vi "SetRef.vi"(8 "error in (no error)":errorcluster, 10 "Set External":bool, 11 "NetA_RSZVL in":refnum<class "NetA_RSZVL.lvclass">) -> (0 "error out":errorcluster, 3 "NetA_RSZVL out":refnum<class "NetA_RSZVL.lvclass">)   [LabVIEW 2014, in "NetA_RSZVL.lvclass"]
uses:
  NetA_RSZVL.lvclass
  NetA_RSZVL.lvclass/NetA_RSZVL.ctl
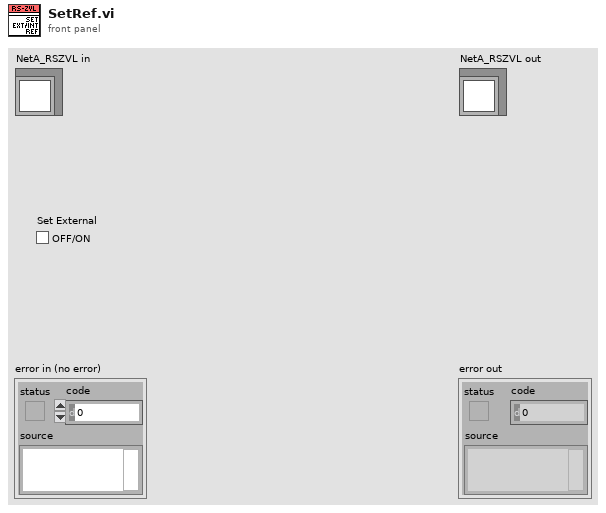
[diagram p1: front panel]
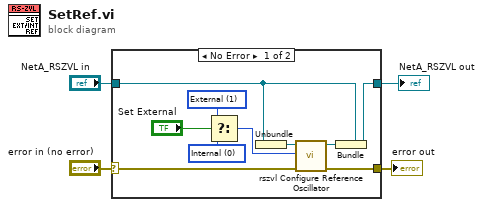
[diagram p0: block diagram]
diagram:
  n1 = case shown="No Error" "error in (no error)" {
    selector: "error in (no error)" -> [w14 w15]
    tunnel: "NetA_RSZVL in" -> [w8 w16]
    tunnel: [w6 w15] -> w2
    tunnel: [w5 w16] -> w1
    frame No Error {
      w11 = 0 items=["Internal", "External"] ("Reference (Internal)")
      w12 = 1 items=["Internal", "External"] ("Reference (Internal)")
      n2 = Select(t=w12, s="Set External", f=w11) -> (s? t:f=w10:i32)
      n3 = Unbundle(w8) -> (w9:refnum<visa-resource-name>)
      n4 = call "rszvl Configure Reference Oscillator.vi"("error in (no error)"=w14, "Reference (Internal)"=w10, "VISA resource name"=w9) -> ("error out"=w6:errorcluster, "VISA resource name out"=w7:refnum<visa-resource-name>)  [unwired: 7 in]
      n5 = Bundle(cluster=w8, w7) -> (w5:refnum<class "NetA_RSZVL.lvclass">)
    }
    frame Error {
    }
  }
  "error out" <- w2
  "NetA_RSZVL out" <- w1
